vi "File Delete.vi"(0 "VISA resource name":refnum<visa-resource-name>, 5 "File Number":u16=1, 11 "error in (no error)":errorcluster) -> (4 "VISA resource name out":refnum<visa-resource-name>, 15 "error out":errorcluster)   [LabVIEW 2020, in "eec EST 300.lvlib"]
doc: "FD <file number>\nDeletes a file from non-volatile memory indicated by the file number."
uses:
  <instrlib>/eec EST 300/eec EST 300.lvlib
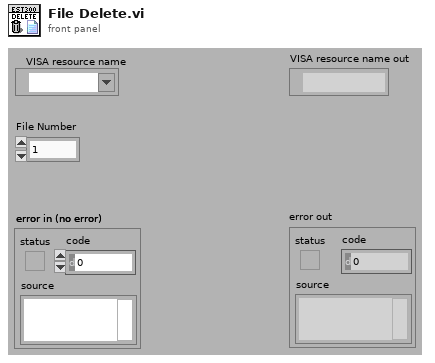
[diagram p1: front panel]
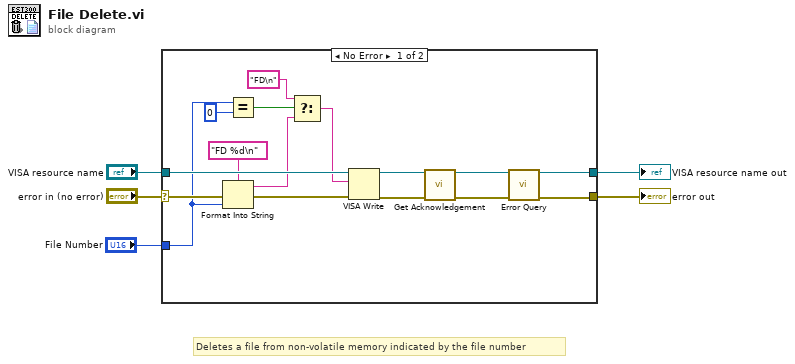
[diagram p0: block diagram]
diagram:
  # "Deletes a file from non-volatile memory indicated by the file number"
  n1 = case shown="No Error" "error in (no error)" {
    selector: "error in (no error)" -> [w17 w23]
    tunnel: [w19 w23] -> w4
    tunnel: [w20 w22] -> w2
    tunnel: "VISA resource name" -> [w21 w22]
    tunnel: "File Number" -> [w11 _]
    frame No Error {
      n2 = Format Into String(format string="FD %d\n" ("\"False\" Command"), error in=w17, w11) -> (resulting string=w7:string, error out=w16:errorcluster)  [unwired: 1 in]
      n3 = Equal?(x=w11, y=u16 0) -> (x = y?=w9:bool)
      n4 = Select(t="FD\n" ("\"False\" Command"), s=w9, f=w7) -> (s? t:f=w6:string)
      n5 = VISA Write(VISA resource name=w21, write buffer=w6, error in (no error)=w16) -> (VISA resource name out=w13:refnum<visa-resource-name>, error out=w12:errorcluster)  [unwired: 1 out]
      n6 = call <instrlib>:"Get Acknowledgement.vi"("VISA resource name"=w13, "error in (no error)"=w12) -> ("VISA resource name out"=w15:refnum<visa-resource-name>, "error out"=w14:errorcluster)  [unwired: 12 in]
      n7 = call <instrlib>:"Error Query.vi"("VISA resource name"=w15, "error in (no error)"=w14) -> ("VISA resource name out"=w20:refnum<visa-resource-name>, "error out"=w19:errorcluster)  [unwired: 10 in, 2 out]
    }
    frame Error {
    }
  }
  "error out" <- w4
  "VISA resource name out" <- w2
